vi "StopSignal-Check.vi"(8 "error in (no error)":errorcluster, 9 "Stop Button":bool, 11 "StopSignal":T1) -> (0 "error out":errorcluster, 1 "Stop?":bool, 2 "Reason":string, 3 "StopSignal(dup)":T1, 4 "timestamp":timestamp)   [LabVIEW 2017, in "StopSignal.lvlib"]
doc: "Check stopsignal is set or not."
uses:
  StopSignal.lvlib
  Typedef/StopSignal.ctl
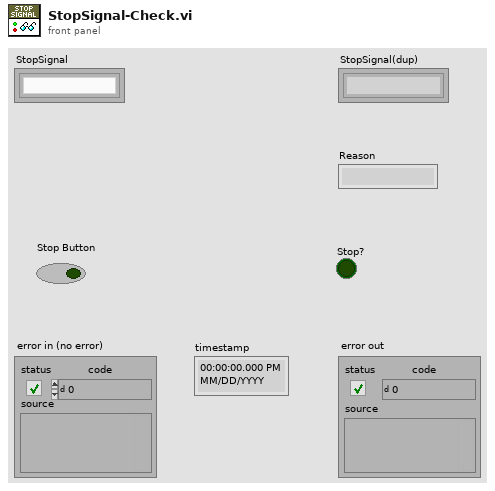
[diagram p1: front panel]
types:
  T1 = typedef "StopSignal.lvlib/StopSignal.ctl" = refnum<k1>
  T2 = typedef "StopSignal.lvlib/Def-StopSignalData.ctl" = cluster{"StopEvent":refnum<user-event>, "StopNotifier":refnum<notifier>, "StopReason":T3}
  T3 = typedef "StopSignal.lvlib/def-StopReason.ctl" = cluster{"Reason":string, "timestamp":timestamp}
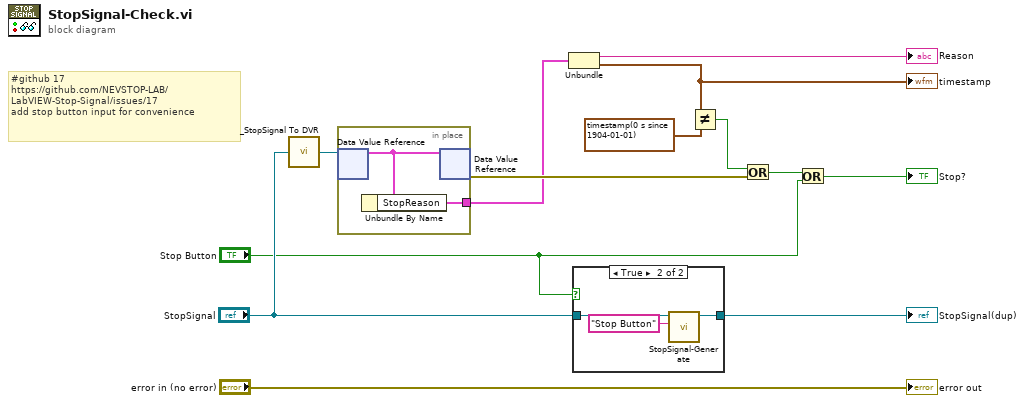
[diagram p0: block diagram]
diagram:
  # "#github 17\nhttps://github.com/NEVSTOP-LAB/LabVIEW-Stop-Signal/issues/17\nadd stop button input for convenience"
  n1 = call "_StopSignal To DVR.vi"("Refnum in"="StopSignal") -> ("Data Value Reference out"=w9:refnum<data-value>)
  n2 = in-place "In Place Element Structure" {
    in-place-border: [w14] -> w5
    n3 = in-place-dvr #1(w9) -> (w15:T2)  [unwired: 1 out]
    n4 = Unbundle By Name(w15) -> ("StopReason"=w14:T3)
    n5 = in-place-dvr #1(w15) -> (w6:errorcluster)  [unwired: 1 out]
  }
  n6 = Unbundle(w5) -> ("Reason"=→"Reason":string, "timestamp"=w11:timestamp)
  "timestamp" <- w11
  n7 = case shown="True" "Stop Button" {
    tunnel: "StopSignal" -> [w16 w19]
    tunnel: [w16 w18] -> w2
    frame False {
    }
    frame True {
      n8 = call "StopSignal-Generate.vi"("reason(\"\")"="Stop Button" ("reason(\"\")"), "StopSignal"=w19) -> ("StopSignal(dup)"=w18:T1)  [unwired: 8 in, 1 out]
    }
  }
  "StopSignal(dup)" <- w2
  n9 = Not Equal?(x=w11, y=timestamp(0 s since 1904-01-01)) -> (x != y?=w7:bool)
  n10 = Or(x=w7, y=w6) -> (x .or. y?=w4:bool)
  n11 = Or(x=w4, y="Stop Button") -> (x .or. y?=→"Stop?":bool)
  "error out" <- "error in (no error)"
